vi "Ethernet-II-Parse.vi"(11 "Input Frame":u8[](array[numeric])=[255, 255, 255, 255, 255, 255, 0, 2, 201, 85, 8, 68, 8, 6, 0, 1, 8, 0, 6, 4, 0, 1, 0, 2, 201, 85, 8, 68, 10, 0, 1, 100, 0, 0, 0, 0, 0, 0, 10, 0, 1, 101, 0, 0, 0, 0, 0, 0, 0, 0, 0, 0, 0, 0, 0, 0, 0, 0, 0, 0, 124, 224, 175, 226] format="%02x") -> (0 "Payload":u8[](array[numeric])=[0, 2, 201, 85, 8, 68, 10, 0, 1, 100, 0, 0, 0, 0, 0, 0, 10, 0, 1, 101, 0, 0, 0, 0, 0, 0, 0, 0, 0, 0, 0, 0, 0, 0, 0, 0, 0, 0] format="%02x", 1 "CRC OK?":bool, 2 "Source MAC":u8[](array[numeric])=[0, 1, 8, 0, 6, 4] format="%02x", 3 "Destination MAC":u8[](array[numeric])=[201, 85, 8, 68, 8, 6] format="%02x", 4 "EtherType":u16=1 format="%04x")   [LabVIEW 2018]
panel:
  out "CRC32Value":u32=2448759633 format="%x"
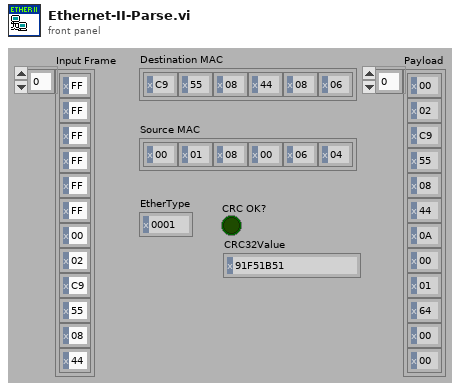
[diagram p1: front panel]
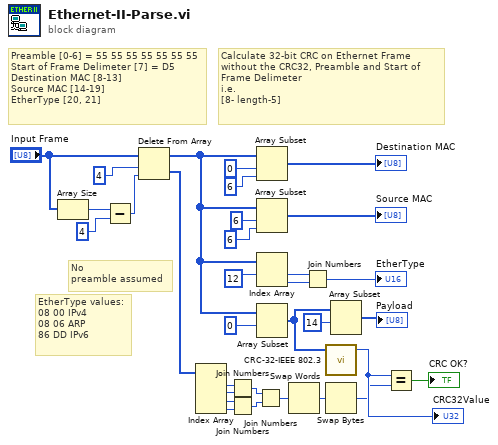
[diagram p0: block diagram]
diagram:
  # "No\npreamble assumed"
  # "EtherType values:\n08 00 IPv4\n08 06 ARP\n86 DD IPv6"
  # "Calculate 32-bit CRC on Ethernet Frame\nwithout the CRC32, Preamble and Start of \nFrame Delimeter\ni.e.\n[8- length-5]"
  # "Preamble [0-6] = 55 55 55 55 55 55 55\nStart of Frame Delimeter [7] = D5\nDestination MAC [8-13]\nSource MAC [14-19]\nEtherType [20, 21]"
  n1 = Array Size(array="Input Frame") -> (size(s)=w27:i32)
  n2 = Subtract(x=w27, y=4) -> (x-y=w31:i32)
  n3 = Delete From Array(array="Input Frame", length=4 ("index"), index=w31) -> (deleted portion=w15:u8[], array with subset deleted=w16:u8[])
  n4 = Index Array(array=w15) -> (element #1=w12:u8, element #2=w11:u8, element #3=w10:u8, element #4=w9:u8)  [unwired: 4 in]
  n5 = Join Numbers(hi=w12, lo=w11) -> ((hi.lo)=w13:u16)
  n6 = Join Numbers(hi=w10, lo=w9) -> ((hi.lo)=w14:u16)
  n7 = Join Numbers(hi=w13, lo=w14) -> ((hi.lo)=w8:u32)
  n8 = Array Subset(array=w16, index=0, length=6) -> (→"Destination MAC":u8[])
  n9 = Array Subset(array=w16, index=6, length=6) -> (→"Source MAC":u8[])
  n10 = Index Array(array=w16, index #1=12 ("index")) -> (element #1=w19:u8, element #2=w18:u8)  [unwired: 1 in]
  n11 = Array Subset(array=w16, index=0) -> (w2:u8[])  [unwired: 1 in]
  n12 = Swap Words(1:w8) -> (0:w7:u32)
  n13 = Join Numbers(hi=w19, lo=w18) -> ((hi.lo)=→"EtherType":u16)
  n14 = call "CRC-32-IEEE 802.3.vi"("Frame in"=w2) -> ("CRC32Value"=w6:u32)  [unwired: 3 in, 1 out]
  "CRC32Value" <- w6
  n15 = Swap Bytes(anything=w7) -> (byte swapped=w5:u32)
  n16 = Array Subset(array=w2, index=14) -> (→"Payload":u8[])  [unwired: 1 in]
  n17 = Equal?(x=w6, y=w5) -> (x = y?=→"CRC OK?":bool)
